vi "Pre Launch Init.vi"(11 "SongQueueActor in":refnum<class "SongQueueActor.lvclass">) -> (0 "error out":errorcluster, 3 "SongQueueActor out":refnum<class "SongQueueActor.lvclass">)   [LabVIEW 2015, in "SongQueueActor.lvlib" / "SongQueueActor.lvclass"]
doc: "(<B>Filename</B>: Actor Framework.lvlib:Actor.lvclass:Pre Launch Init.vi)\n\nDefines behavior that occurs after the Launch Nested Actor method is invoked but before the actor's Actor Core method begins running.\n\nBy default, this method does nothing. A descendant class may override it to define behavior."
uses:
  SongQueueActor.lvclass
  SongQueueActor.lvclass/SongQueueActor.ctl
  <vilib>/ActorFramework/Actor/Actor.lvclass
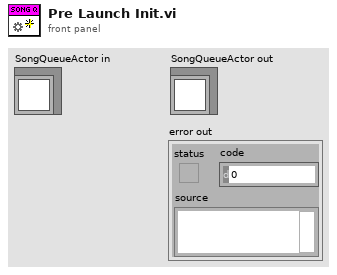
[diagram p1: front panel]
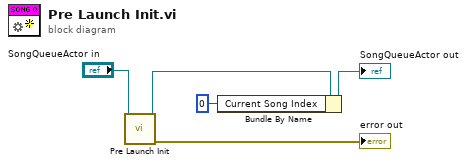
[diagram p0: block diagram]
diagram:
  n1 = call-parent "Pre Launch Init.vi"("Actor in"="SongQueueActor in") -> ("error out"=→"error out":errorcluster, "Actor out"=w3:refnum<class "SongQueueActor.lvclass">)  [unwired: 9 in]
  n2 = Bundle By Name(cluster=w3, "Current Song Index"=0) -> (→"SongQueueActor out":refnum<class "SongQueueActor.lvclass">)
